vi "GetRampTable.vi"(8 "error in (no error)":errorcluster, 11 "RampProgramModel in":refnum<class "RampProgramModel.lvclass">) -> (0 "error out":errorcluster, 2 "RampTable":string[][](array[string]), 3 "RampProgramModel out":refnum<class "RampProgramModel.lvclass">)   [LabVIEW 2013, in "RampProgramModel.lvclass"]
uses:
  RampProgramModel.lvclass
  RampProgramModel.lvclass/RampProgramModel.ctl
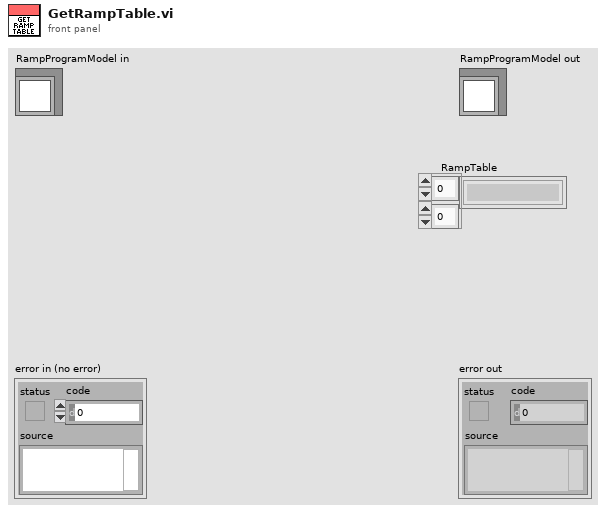
[diagram p1: front panel]
types:
  T1 = cluster{"SP (°C)":dbl, "Cooling rate (°C/min)":dbl, "Dwell Time @ SP (sec)":u32}[]
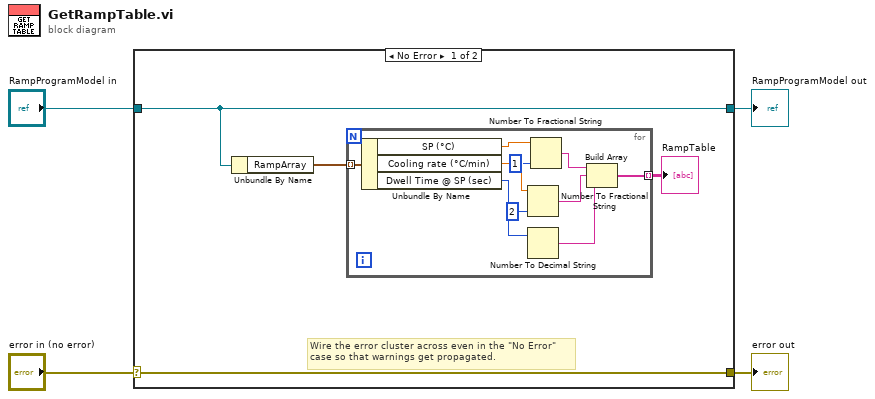
[diagram p0: block diagram]
diagram:
  n1 = case shown="No Error" "error in (no error)" {
    selector: "error in (no error)" -> [w8 w20]
    tunnel: [w8 w20] -> w3
    tunnel: [w7 w19] -> w1
    tunnel: "RampProgramModel in" -> [w7 w19]
    frame No Error {
      # "Wire the error cluster across even in the \"No Error\"\ncase so that warnings get propagated."
      n2 = Unbundle By Name(w7) -> ("RampArray"=w6:T1)
      n3 = for {
        tunnel: w6 -> [w18] mode=indexing
        tunnel: [w11] -> w5 mode=indexing
        n4 = Unbundle By Name(w18) -> ("SP (°C)"=w15:dbl, "Cooling rate (°C/min)"=w16:dbl, "Dwell Time @ SP (sec)"=w17:u32)
        n5 = Number To Fractional String(number=w16, precision (6)=i16 2) -> (F-format string=w13:string)  [unwired: 2 in]
        n6 = Number To Decimal String(number=w17) -> (decimal integer string=w12:string)  [unwired: 1 in]
        n7 = Number To Fractional String(number=w15, precision (6)=i16 1) -> (F-format string=w14:string)  [unwired: 2 in]
        n8 = Build Array(w14, w13, w12) -> (w11:string[])
      }
      "RampTable" <- w5
    }
    frame Error {
    }
  }
  "error out" <- w3
  "RampProgramModel out" <- w1
